vi "HighSpeedInit.vi"(8 "error in":errorcluster, 10 "Fast":bool=TRUE, 11 "VISA Refnum in":refnum<visa-resource-name>) -> (0 "error out":errorcluster, 3 "VISA Refnum out":refnum<visa-resource-name>)   [LabVIEW 2017]
uses:
  <vilib>/Instr/_visa.llb/VISA Configure Serial Port (Instr).vi
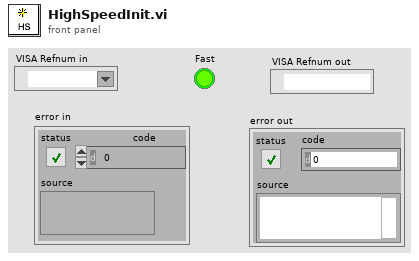
[diagram p1: front panel]
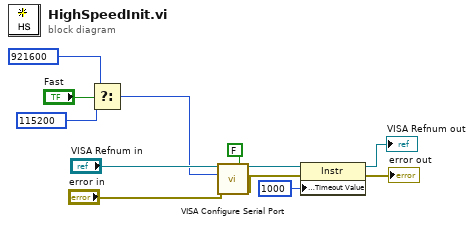
[diagram p0: block diagram]
diagram:
  n1 = Select(t=u32 921600 ("baud rate (115200)"), s="Fast", f=u32 115200 ("baud rate (115200)")) -> (s? t:f=w1:u32)
  n2 = call-poly "VISA Configure Serial Port"("VISA resource name"="VISA Refnum in", "Enable Termination\nChar (T)"=FALSE ("Enable Termination\nChar (T)"), "baud rate (9600)"=w1, "error in (no error)"="error in") -> ("VISA resource name out"=w11:refnum<visa-resource-name>, "error out"=w6:errorcluster)  [unwired: 10 in]
  n3 = property class="Instr"(reference=w11, error in=w6, "General Settings:Timeout Value"=u32 1000) -> (reference out=→"VISA Refnum out":refnum<visa-resource-name>, error out=→"error out":errorcluster)
